vi "milliGAT Configure and Run Continuous - Parallel Different VISA.vi"() -> ()   [LabVIEW 2015]
uses:
  Global FIA milliGAT.lvlib
  Public/Utility/Pump Direction.ctl
  Public/Utility/Pump Address.ctl
panel:
  out "error out closing 2":errorcluster
  out "error out closing 1":errorcluster
  in  "VISA resource name 2":refnum<visa-resource-name>="COM18"
  in  "Flow Parameters 2":T1={"Peak Flow (uL/s)"=1.0, "Starting Flow (uL/s)"=0.1, "Acceleration (uL/s^2)"=500.0, "Deceleration (uL/s^2)"=500.0}
  in  "Pump ID (0:A) 2":T2=enum."B"
  out "Microliters 2":dbl
  in  "Direction 2":T3=enum."Dispense"
  in  "Serial Configuration 2":cluster{"Baud Rate":u32}={"Baud Rate"=9600} {"Baud Rate" items=["300"=300, "600"=600, "1200"=1200, "2400"=2400, "4800"=4800, "9600"=9600, "19200"=19200]}
  out "error out 2":errorcluster
  in  "Flow Parameters":T1={"Peak Flow (uL/s)"=0.5, "Starting Flow (uL/s)"=0.1, "Acceleration (uL/s^2)"=500.0, "Deceleration (uL/s^2)"=500.0}
  in  "Pump ID (0:A)":T2
  in  "Stop":bool
  out "Microliters":dbl
  in  "Direction":T3=enum."Dispense"
  in  "Serial Configuration":cluster{"Baud Rate":u32}={"Baud Rate"=9600} {"Baud Rate" items=["300"=300, "600"=600, "1200"=1200, "2400"=2400, "4800"=4800, "9600"=9600, "19200"=19200]}
  out "error out":errorcluster
  in  "VISA resource name":refnum<visa-resource-name>="COM16"
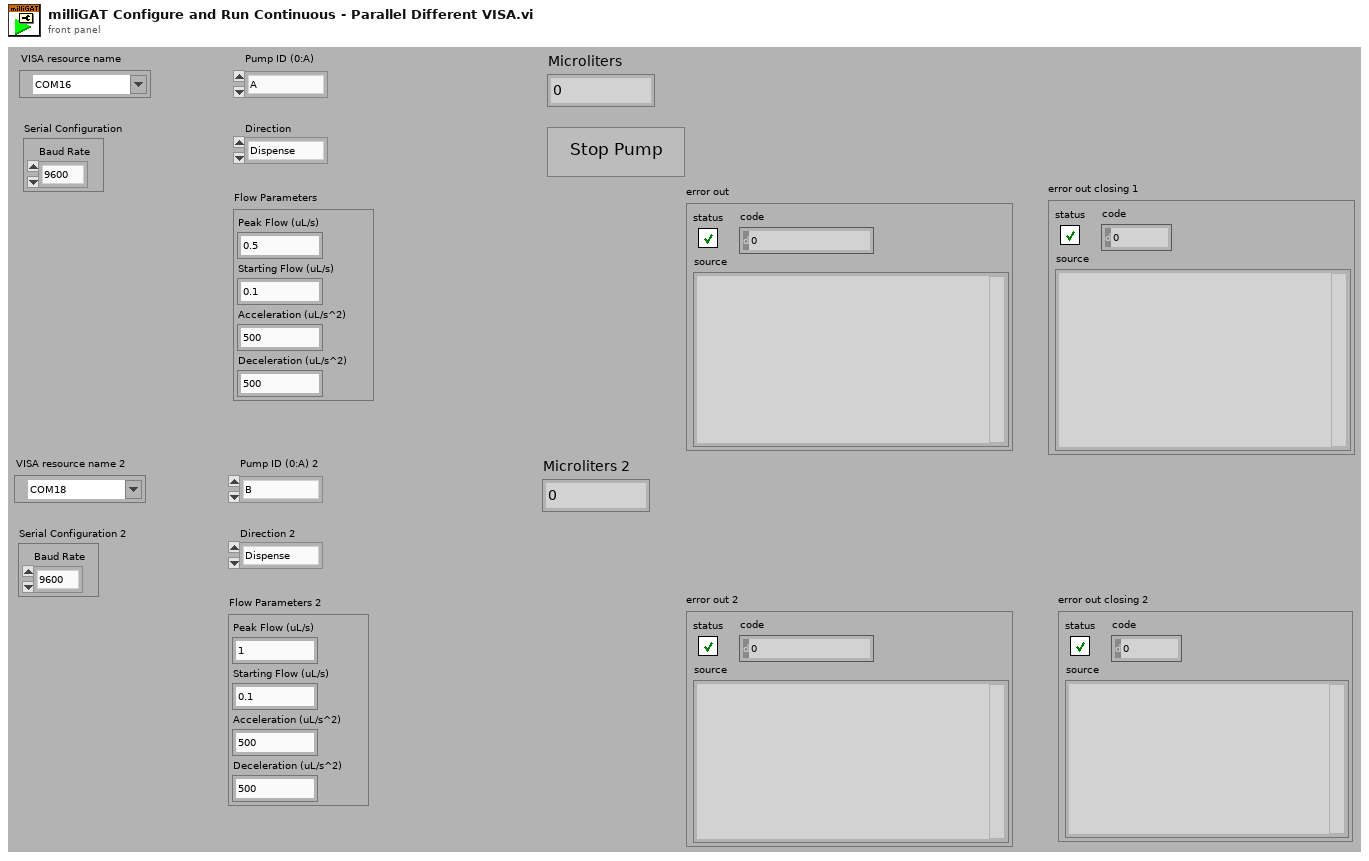
[diagram p1: front panel]
types:
  T1 = cluster{"Peak Flow (uL/s)":dbl, "Starting Flow (uL/s)":dbl, "Acceleration (uL/s^2)":dbl, "Deceleration (uL/s^2)":dbl}
  T2 = typedef "Global FIA milliGAT.lvlib/Pump Address.ctl" = enum16{"A", "B", "C", "D", "E", "F", "G", "H", "I", "J", "K", "L", "M", "N", "O", "P", "Q", "R", "S", "T", "U", "V", "W", "X", "Y", "Z", "a", "b", "c", "d", "e", "f", "g", "h", "i", "j", "k", "l", "m", "n", "o", "p", "q", "r", "s", "t", "u", "v", "w", "x", "y", "z", "0", "1", "2", "3", "4", "5", "6", "7", "8", "9"}
  T3 = typedef "Global FIA milliGAT.lvlib/Pump Direction.ctl" = enum16{"Aspirate", "Dispense"}
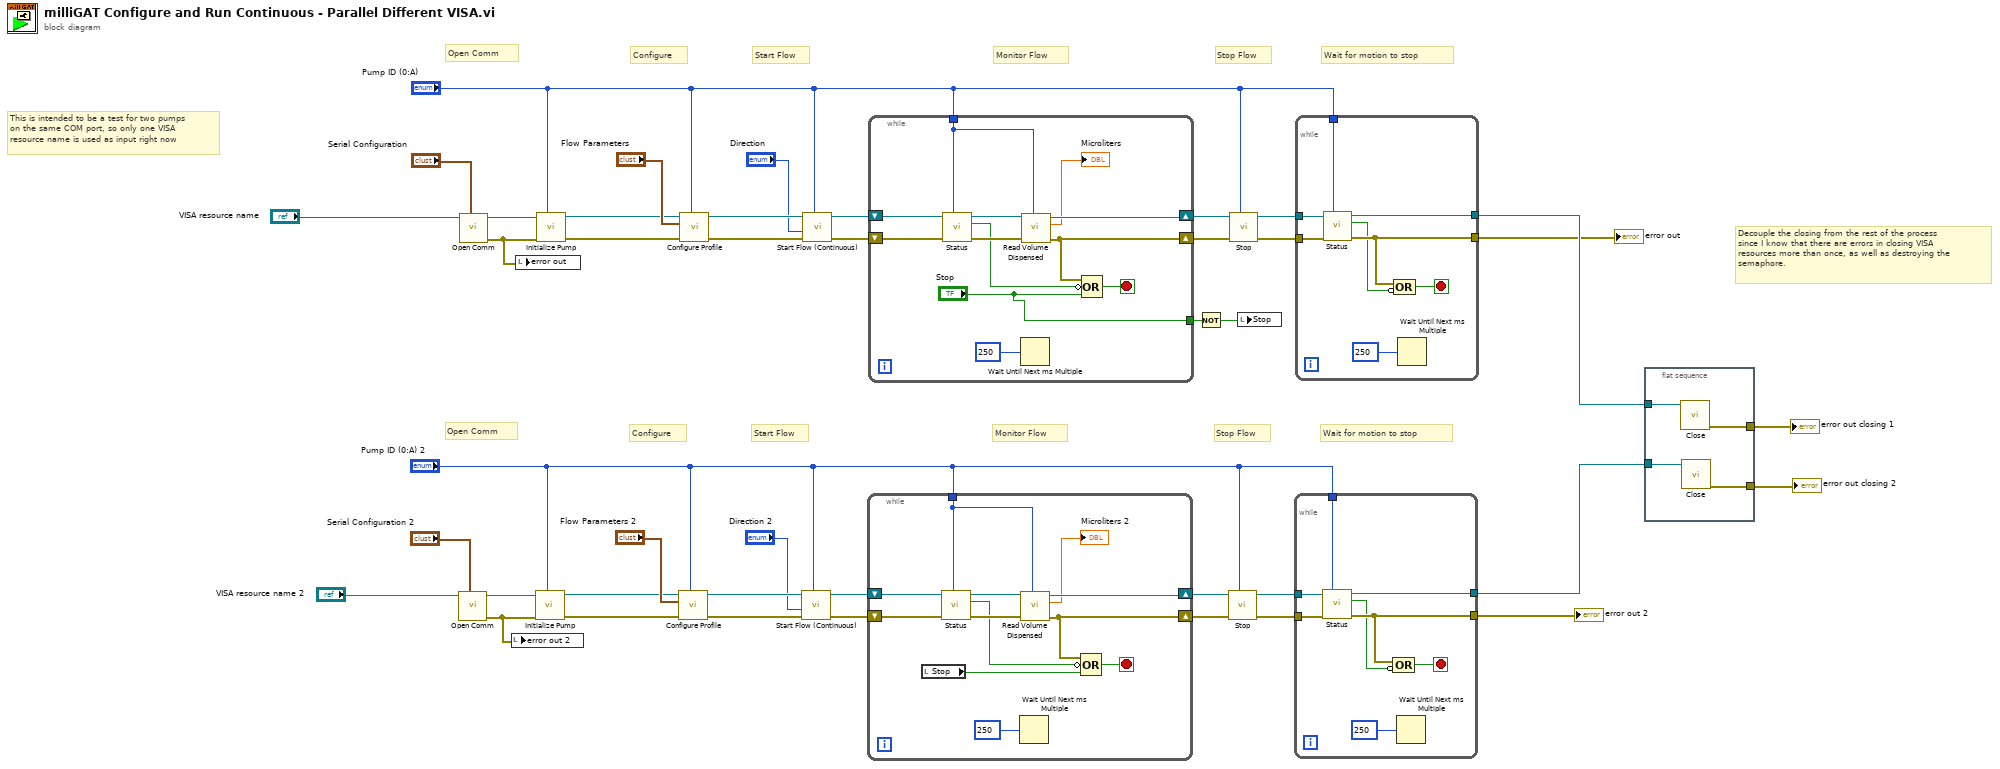
[diagram p0: block diagram]
diagram:
  # "Decouple the closing from the rest of the process\nsince I know that there are errors in closing VISA\nresources more than once, as well as destroying the\nsemaphore."
  # "This is intended to be a test for two pumps\non the same COM port, so only one VISA\nresource name is used as input right now"
  # "Stop Flow"
  # "Open Comm"
  # "Start Flow"
  # "Configure"
  # "Monitor Flow"
  # "Wait for motion to stop"
  # "Stop Flow"
  # "Open Comm"
  # "Start Flow"
  # "Configure"
  # "Monitor Flow"
  # "Wait for motion to stop"
  n1 = call "Open Comm.vi"("Serial Configuration"="Serial Configuration 2", "VISA resource in"="VISA resource name 2") -> ("error out"=w14:errorcluster, "VISA resource out"=w20:refnum<visa-resource-name>)  [unwired: 8 in]
  n2 = call "Open Comm.vi"("Serial Configuration"="Serial Configuration", "VISA resource in"="VISA resource name") -> ("error out"=w30:errorcluster, "VISA resource out"=w36:refnum<visa-resource-name>)  [unwired: 8 in]
  n3 = local write "error out 2"(w14) -> ()
  n4 = local write "error out"(w30) -> ()
  n5 = call "Initialize Pump.vi"("Pump ID (0:A)"="Pump ID (0:A) 2", "error in (no error)"=w14, "VISA resource in"=w20) -> ("error out"=w11:errorcluster, "VISA resource out"=w12:refnum<visa-resource-name>)  [unwired: 7 in]
  n6 = call "Initialize Pump.vi"("Pump ID (0:A)"="Pump ID (0:A)", "error in (no error)"=w30, "VISA resource in"=w36) -> ("error out"=w27:errorcluster, "VISA resource out"=w28:refnum<visa-resource-name>)  [unwired: 7 in]
  n7 = call "Configure Profile.vi"("Pump ID (0:A)"="Pump ID (0:A) 2", "error in (no error)"=w11, "Flow Parameters"="Flow Parameters 2", "VISA resource in"=w12) -> ("error out"=w25:errorcluster, "VISA resource out"=w26:refnum<visa-resource-name>)  [unwired: 6 in]
  n8 = call "Configure Profile.vi"("Pump ID (0:A)"="Pump ID (0:A)", "error in (no error)"=w27, "Flow Parameters"="Flow Parameters", "VISA resource in"=w28) -> ("error out"=w41:errorcluster, "VISA resource out"=w42:refnum<visa-resource-name>)  [unwired: 6 in]
  n9 = call "Start Flow (Continuous).vi"("Pump ID (0:A)"="Pump ID (0:A) 2", "error in (no error)"=w25, "Direction (0:Aspirate)"="Direction 2", "VISA resource in"=w26) -> ("error out"=w22:errorcluster, "VISA resource out"=w23:refnum<visa-resource-name>)  [unwired: 6 in]
  n10 = call "Start Flow (Continuous).vi"("Pump ID (0:A)"="Pump ID (0:A)", "error in (no error)"=w41, "Direction (0:Aspirate)"="Direction", "VISA resource in"=w42) -> ("error out"=w38:errorcluster, "VISA resource out"=w39:refnum<visa-resource-name>)  [unwired: 6 in]
  n11 = while {
    shift-right: [w54] -> w17
    shift-left: w23 -> [w52]
    tunnel: "Pump ID (0:A) 2" -> [w51]
    shift-right: [w45] -> w18
    shift-left: w22 -> [w53]
    stop <- w46 stop-if-true
    n12 = local read "Stop"() -> (w43:bool)
    n13 = call "Status.vi"("Pump ID (0:A)"=w51, "error in (no error)"=w53, "VISA resource in"=w52) -> ("error out"=w48:errorcluster, "moving"=w44:bool, "VISA resource out"=w49:refnum<visa-resource-name>)  [unwired: 6 in]
    n14 = Wait Until Next ms Multiple(millisecond multiple=u32 250) -> ()  [unwired: 1 out]
    n15 = call "Read Volume Dispensed.vi"("Pump ID (0:A)"=w51, "error in (no error)"=w48, "VISA resource in"=w49) -> ("error out"=w45:errorcluster, "microliters"=→"Microliters 2":dbl, "VISA resource out"=w54:refnum<visa-resource-name>)  [unwired: 6 in]
    n16 = Compound Arithmetic op=OR(w45, invert w44, w43) -> (w46:bool)
  }
  n17 = while {
    shift-right: [w66] -> w33
    shift-left: w39 -> [w64]
    tunnel: "Pump ID (0:A)" -> [w63]
    shift-right: [w57] -> w34
    shift-left: w38 -> [w65]
    tunnel: ["Stop"] -> w2
    stop <- w58 stop-if-true
    n18 = call "Status.vi"("Pump ID (0:A)"=w63, "error in (no error)"=w65, "VISA resource in"=w64) -> ("error out"=w60:errorcluster, "moving"=w56:bool, "VISA resource out"=w61:refnum<visa-resource-name>)  [unwired: 6 in]
    n19 = Wait Until Next ms Multiple(millisecond multiple=u32 250) -> ()  [unwired: 1 out]
    n20 = call "Read Volume Dispensed.vi"("Pump ID (0:A)"=w63, "error in (no error)"=w60, "VISA resource in"=w61) -> ("error out"=w57:errorcluster, "microliters"=→"Microliters":dbl, "VISA resource out"=w66:refnum<visa-resource-name>)  [unwired: 6 in]
    n21 = Compound Arithmetic op=OR(w57, invert w56, "Stop") -> (w58:bool)
  }
  n22 = Not(x=w2) -> (.not. x?=w1:bool)
  n23 = call "Stop.vi"("Pump ID (0:A)"="Pump ID (0:A) 2", "error in (no error)"=w18, "VISA resource in"=w17) -> ("error out"=w16:errorcluster, "VISA resource out"=w15:refnum<visa-resource-name>)  [unwired: 7 in]
  n24 = call "Stop.vi"("Pump ID (0:A)"="Pump ID (0:A)", "error in (no error)"=w34, "VISA resource in"=w33) -> ("error out"=w32:errorcluster, "VISA resource out"=w31:refnum<visa-resource-name>)  [unwired: 7 in]
  n25 = local write "Stop"(w1) -> ()
  n26 = while {
    tunnel: w16 -> [w73]
    tunnel: w15 -> [w74]
    tunnel: "Pump ID (0:A) 2" -> [w72]
    tunnel: [w70] -> w5
    tunnel: [w71] -> w7
    stop <- w68 stop-if-true
    n27 = call "Status.vi"("Pump ID (0:A)"=w72, "error in (no error)"=w73, "VISA resource in"=w74) -> ("error out"=w70:errorcluster, "moving"=w69:bool, "VISA resource out"=w71:refnum<visa-resource-name>)  [unwired: 6 in]
    n28 = Compound Arithmetic op=OR(w70, invert w69) -> (w68:bool)
    n29 = Wait Until Next ms Multiple(millisecond multiple=u32 250) -> ()  [unwired: 1 out]
  }
  "error out 2" <- w5
  n30 = while {
    tunnel: w32 -> [w81]
    tunnel: w31 -> [w82]
    tunnel: "Pump ID (0:A)" -> [w80]
    tunnel: [w78] -> w6
    tunnel: [w79] -> w8
    stop <- w76 stop-if-true
    n31 = call "Status.vi"("Pump ID (0:A)"=w80, "error in (no error)"=w81, "VISA resource in"=w82) -> ("error out"=w78:errorcluster, "moving"=w77:bool, "VISA resource out"=w79:refnum<visa-resource-name>)  [unwired: 6 in]
    n32 = Compound Arithmetic op=OR(w78, invert w77) -> (w76:bool)
    n33 = Wait Until Next ms Multiple(millisecond multiple=u32 250) -> ()  [unwired: 1 out]
  }
  "error out" <- w6
  n34 = flat-sequence {
    tunnel: w8 -> [w86]
    tunnel: w7 -> [w85]
    tunnel: [w84] -> w4
    tunnel: [w83] -> w3
    frame #0 {
      n35 = call "Close.vi"("VISA resource in"=w86) -> ("error out"=w84:errorcluster)  [unwired: 10 in]
      n36 = call "Close.vi"("VISA resource in"=w85) -> ("error out"=w83:errorcluster)  [unwired: 10 in]
    }
  }
  "error out closing 1" <- w4
  "error out closing 2" <- w3
